vi "actuatorSelect.vi"(8 "error in (no error)":errorcluster, 11 "Devices":u32) -> (0 "error out":errorcluster, 3 "Selected":u32)   [LabVIEW 2019]
doc: "Allows user to select the actuator to communicate with. Currently supports up to 6 actuators.\n\nWritten by: Complete Automated Solutions\nwww.CompleteAutomatedSolutions.com"
panel:
  in  "continue":bool caption="Continue"
  in  "acutator":T1(ring) caption="Select Acutator"
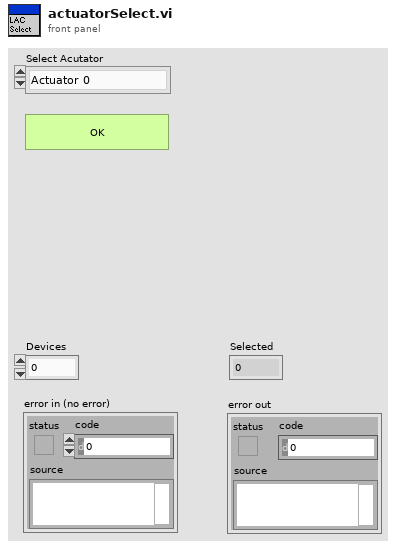
[diagram p1: front panel]
types:
  T1 = enum16{"Actuator 0", "Actuator 1", "Actuator 2", "Actuator 3", "Actuator 4", "Actuator 5"}
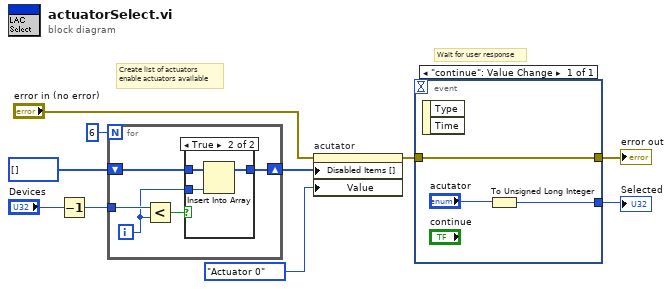
[diagram p0: block diagram]
diagram:
  # "Wait for user response"
  # "Create list of actuators\nenable actuators available"
  n1 = Decrement(x="Devices") -> (x-1=w6:u32)
  n2 = for {
    N: 6 -> [_]
    tunnel: w6 -> [w12]
    shift-right: [w13] -> w8
    shift-left: i32[] [] ("Disabled Items []") -> [w14]
    i -> [w11]
    n3 = Less?(x=w12, y=w11) -> (x < y?=w15:bool)
    n4 = case shown="True" w15 {
      tunnel: w14 -> [w16 w19]
      tunnel: [w16 w18] -> w13
      tunnel: w11 -> [_ w17]
      frame False {
      }
      frame True {
        n5 = Insert Into Array(array=w19, new element=w17) -> (w18:i32[])  [unwired: 1 in]
      }
    }
  }
  n6 = property on="acutator" class="Enum (strict)"(error in="error in (no error)", "Disabled Items []"=w8, "Value"=T1."Actuator 0" ("acutator")) -> (error out=w4:errorcluster)  [unwired: 1 in, 1 out]
  n7 = event shown="[0] \"continue\": Value Change" {
    selector: _ -> [_]
    dyn-events: _ -> [_]
    timeout: _ -> [_]
    tunnel: w4 -> [w20]
    tunnel: [w21] -> w3
    tunnel: [w20] -> w2
    event "continue": Value Change {
      n8 = event-data() -> ()  [unwired: 3 out]
      n9 = To Unsigned Long Integer(number="acutator") -> (unsigned 32bit integer=w21:u32)
    }
  }
  "Selected" <- w3
  "error out" <- w2
